vi "GetMachineName.vi"() -> (2 "ComputerName":string)   [LabVIEW 2022 SP3]
uses:
  <vilib>/Utility/error.llb/Trim Whitespace One-Sided.vi
  kernel32.dll
panel:
  # "Obtains a name for this machine, either from Windows kernel, or, on other platforms, the first componrent of \"hostname\""
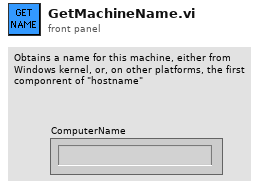
[diagram p1: front panel]
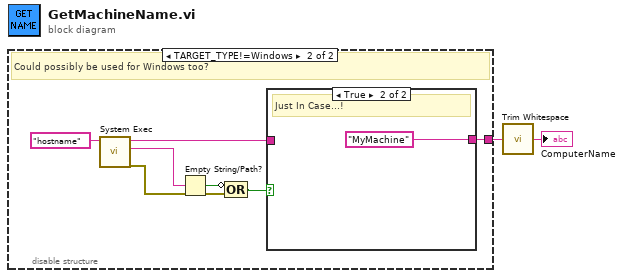
[diagram p0: block diagram]
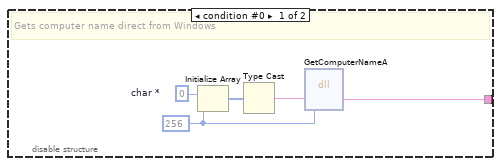
[diagram p2: hidden frame]
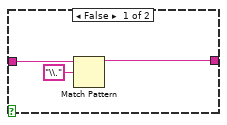
[diagram p3: hidden frame]
diagram:
  n1 = disable-structure shown="TARGET_TYPE!=Windows" {
    disable-tunnel: [w3 w12] -> w2
    frame condition #0 {
      w7 = 256 ("dimension size")
      w4 = u8 0  # char *
      # "Gets computer name direct from Windows"
      n2 = Initialize Array(w4, w7) -> (w5:u8[])
      n3 = Type Cast(x=w5) -> (*(type *) &x=w6:string)  [unwired: 1 in]
      n4 = dll-call lib="kernel32.dll" fn="GetComputerNameA" label="unsigned long GetComputerNameA(CStr lpBuffer, long *nSize);"("lpBuffer"=w6, "nSize"=w7) -> ("lpBuffer"=w3:string)  [unwired: 5 in, 2 out]
    }
    frame condition #1 (active) {
      # "Could possibly be used for Windows too?"
      n5 = call <vilib>:"System Exec.vi"("command line"="hostname") -> ("error out"=w8:errorcluster, "standard error"=w11:string, "standard output"=w13:string)  [unwired: 7 in, 1 out]
      n6 = Empty String/Path?(string/path=w11) -> (empty?=w9:bool)
      n7 = Compound Arithmetic op=OR(invert w9, w8) -> (w10:bool)
      n8 = case shown="True" w10 {
        tunnel: w13 -> [w17 _]
        tunnel: [w15 "MyMachine" ("standard output")] -> w12
        frame False {
          n9 = Match Pattern(string=w17, regular expression="\\.") -> (before substring=w15:string)  [unwired: 1 in, 3 out]
        }
        frame True {
          # "Just In Case...!"
        }
      }
    }
  }
  n10 = call <vilib>:"Trim Whitespace.vi"("string"=w2) -> ("trimmed string"=→"ComputerName":string)  [unwired: 1 in]
